vi "CRYGet All DataView Graph Ref.vi"(11 "DataViewb in":T1) -> (0 "Graph VIRef Out":refnum<vi>[](array[refnum]), 3 "sName Array Out":string)   [LabVIEW 2013]
uses:
  Control/Graph Main Info Cluster.ctl
  Control/SplitterBar.ctl
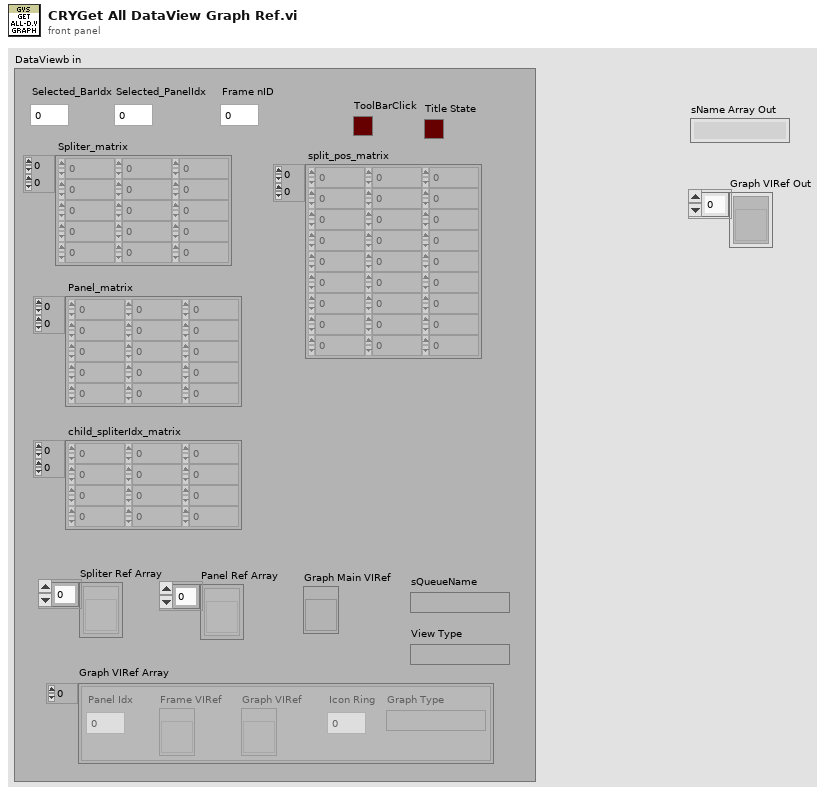
[diagram p1: front panel]
types:
  T1 = typedef "Graph Main Info Cluster.ctl" = cluster{"Selected_BarIdx":i32, "Selected_PanelIdx":i32, "Graph Main VIRef":refnum<vi>, "ToolBarClick":bool, "Spliter Ref Array":refnum<vi>[], "Panel Ref Array":refnum<vi>[], "Spliter_matrix":i32[][], "Panel_matrix":i32[][], "child_spliterIdx_matrix":i32[][], "split_pos_matrix":i32[][], "Title State":bool, "sQueueName":string, "Frame nID":i32, "Graph VIRef Array":cluster{"Graph VIRef":refnum<vi>, "Panel Idx":i32, "Frame VIRef":refnum<vi>, "Icon Ring":i32, "Graph Type":string}[], "View Type":string}
  T2 = cluster{"Graph VIRef":refnum<vi>, "Panel Idx":i32, "Frame VIRef":refnum<vi>, "Icon Ring":i32, "Graph Type":string}[]
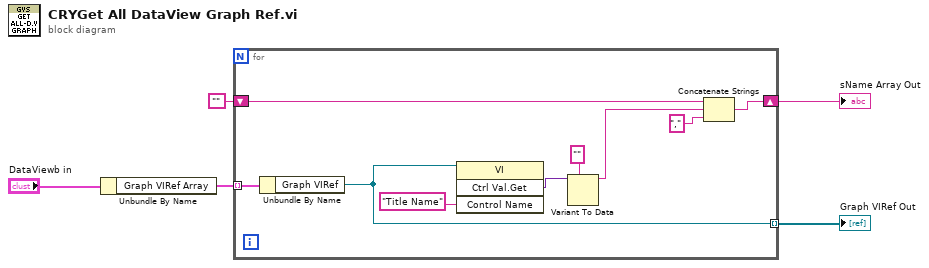
[diagram p0: block diagram]
diagram:
  n1 = Unbundle By Name("DataViewb in") -> ("Graph VIRef Array"=w1:T2)
  n2 = for {
    shift-right: [w12] -> w2
    shift-left: "" -> [w13]
    tunnel: [w6] -> w3 mode=indexing
    tunnel: w1 -> [w7] mode=indexing
    n3 = Unbundle By Name(w7) -> ("Graph VIRef"=w6:refnum<vi>)
    n4 = invoke class="VI" method="Ctrl Val.Get"(reference=w6, "Control Name"="Title Name" ("Label Name")) -> ("Get Control Value Variant"=w10:variant)  [unwired: 2 in, 3 out]
    n5 = Variant To Data(type="" ("string"), Variant=w10) -> (data=w8:string)  [unwired: 1 in, 1 out]
    n6 = Concatenate Strings(w13, w8, "," ("string")) -> (w12:string)
  }
  "Graph VIRef Out" <- w3
  "sName Array Out" <- w2
